vi "SEVEN SEGMENT DISPLAY FROM 0-25.vi"() -> ()   [LabVIEW 2019]
panel:
  in  "STOP":bool
  in  "NUMBER":u8
  out "E 2":bool
  out "D 2":bool
  out "C 2":bool
  out "F 2":bool
  out "G 2":bool
  out "B 2":bool
  out "A 2":bool
  out "E":bool
  out "D":bool
  out "C":bool
  out "F":bool
  out "G":bool
  out "B":bool
  out "A":bool
  # "SEVEN SEGMENT DISPLAY FROM 0-25"
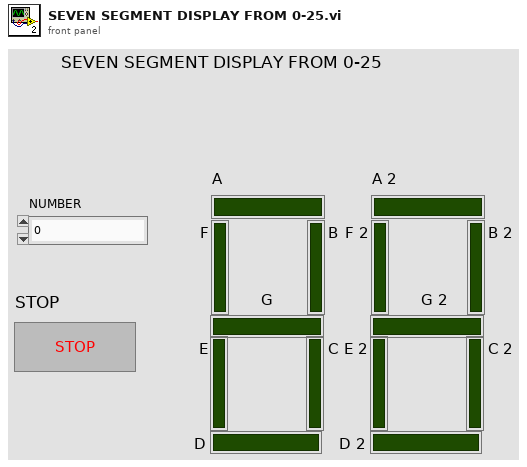
[diagram p1: front panel]
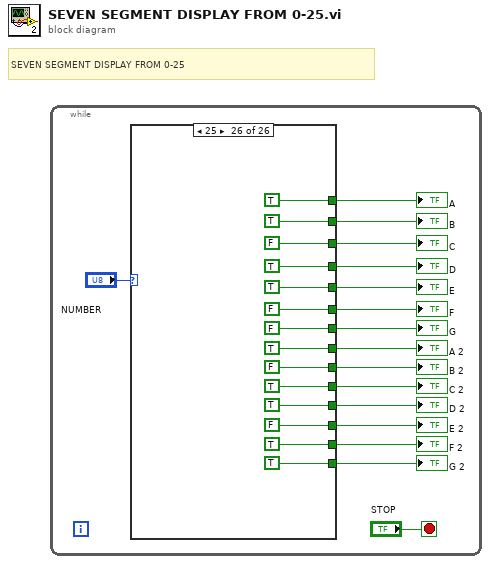
[diagram p0: block diagram]
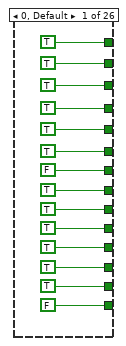
[diagram p2: hidden frame]
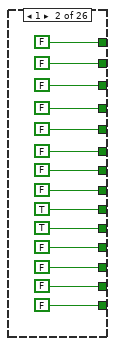
[diagram p3: hidden frame]
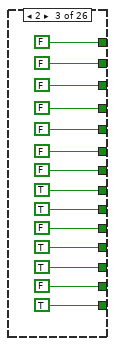
[diagram p4: hidden frame]
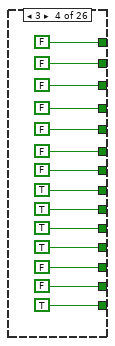
[diagram p5: hidden frame]
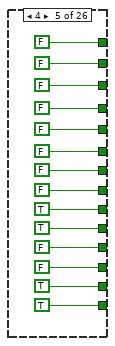
[diagram p6: hidden frame]
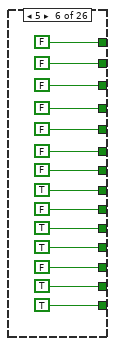
[diagram p7: hidden frame]
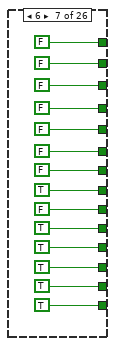
[diagram p8: hidden frame]
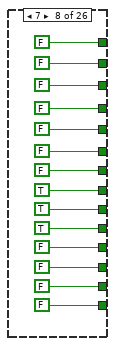
[diagram p9: hidden frame]
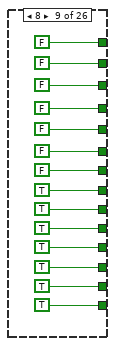
[diagram p10: hidden frame]
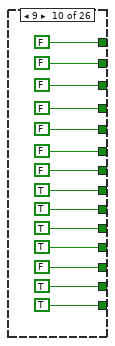
[diagram p11: hidden frame]
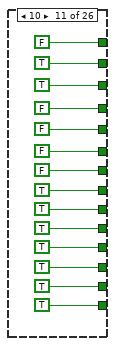
[diagram p12: hidden frame]
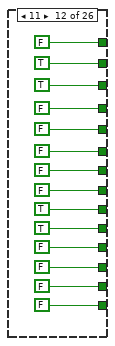
[diagram p13: hidden frame]
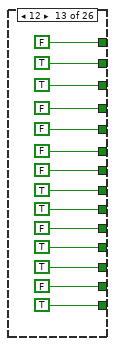
[diagram p14: hidden frame]
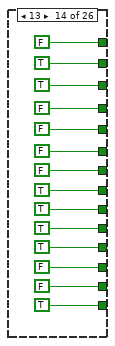
[diagram p15: hidden frame]
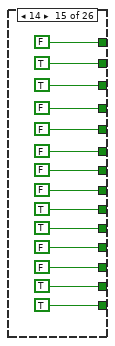
[diagram p16: hidden frame]
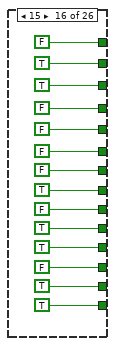
[diagram p17: hidden frame]
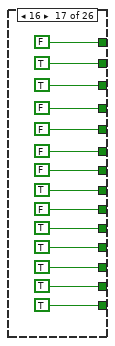
[diagram p18: hidden frame]
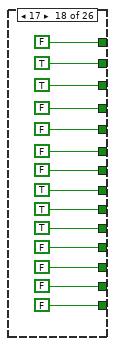
[diagram p19: hidden frame]
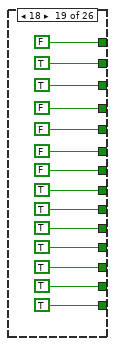
[diagram p20: hidden frame]
diagram:
  # "SEVEN SEGMENT DISPLAY FROM 0-25"
  n1 = while {
    stop <- "STOP" stop-if-true
    n2 = case shown="25" "NUMBER" {
      tunnel: [TRUE ("A") FALSE ("A") FALSE ("A") FALSE ("A") FALSE ("A") FALSE ("A") FALSE ("A") FALSE ("A") FALSE ("A") FALSE ("A") FALSE ("A") FALSE ("A") FALSE ("A") FALSE ("A") FALSE ("A") FALSE ("A") FALSE ("A") FALSE ("A") FALSE ("A") FALSE ("A") TRUE ("A") TRUE ("A") TRUE ("A") TRUE ("A") TRUE ("A") TRUE ("A")] -> w16
      tunnel: [FALSE ("G") FALSE ("G") FALSE ("G") FALSE ("G") FALSE ("G") FALSE ("G") FALSE ("G") FALSE ("G") FALSE ("G") FALSE ("G") FALSE ("G") FALSE ("G") FALSE ("G") FALSE ("G") FALSE ("G") FALSE ("G") FALSE ("G") FALSE ("G") FALSE ("G") FALSE ("G") TRUE ("G") FALSE ("G") FALSE ("G") FALSE ("G") FALSE ("G") FALSE ("G")] -> w15
      tunnel: [TRUE ("F") FALSE ("F") FALSE ("F") FALSE ("F") FALSE ("F") FALSE ("F") FALSE ("F") FALSE ("F") FALSE ("F") FALSE ("F") FALSE ("F") FALSE ("F") FALSE ("F") FALSE ("F") FALSE ("F") FALSE ("F") FALSE ("F") FALSE ("F") FALSE ("F") FALSE ("F") FALSE ("F") FALSE ("F") FALSE ("F") FALSE ("F") FALSE ("F") FALSE ("F")] -> w14
      tunnel: [TRUE ("C") FALSE ("C") FALSE ("C") FALSE ("C") FALSE ("C") FALSE ("C") FALSE ("C") FALSE ("C") FALSE ("C") FALSE ("C") TRUE ("C") TRUE ("C") TRUE ("C") TRUE ("C") TRUE ("C") TRUE ("C") TRUE ("C") TRUE ("C") TRUE ("C") TRUE ("C") FALSE ("C") FALSE ("C") FALSE ("C") FALSE ("C") FALSE ("C") FALSE ("C")] -> w13
      tunnel: [TRUE ("D") FALSE ("D") FALSE ("D") FALSE ("D") FALSE ("D") FALSE ("D") FALSE ("D") FALSE ("D") FALSE ("D") FALSE ("D") FALSE ("D") FALSE ("D") FALSE ("D") FALSE ("D") FALSE ("D") FALSE ("D") FALSE ("D") FALSE ("D") FALSE ("D") FALSE ("D") TRUE ("D") TRUE ("D") TRUE ("D") TRUE ("D") TRUE ("D") TRUE ("D")] -> w12
      tunnel: [TRUE ("E") FALSE ("E") FALSE ("E") FALSE ("E") FALSE ("E") FALSE ("E") FALSE ("E") FALSE ("E") FALSE ("E") FALSE ("E") FALSE ("E") FALSE ("E") FALSE ("E") FALSE ("E") FALSE ("E") FALSE ("E") FALSE ("E") FALSE ("E") FALSE ("E") FALSE ("E") TRUE ("E") TRUE ("E") TRUE ("E") TRUE ("E") TRUE ("E") TRUE ("E")] -> w11
      tunnel: [TRUE ("A 2") FALSE ("A 2") TRUE ("A 2") TRUE ("A 2") FALSE ("A 2") TRUE ("A 2") TRUE ("A 2") TRUE ("A 2") TRUE ("A 2") TRUE ("A 2") TRUE ("A 2") FALSE ("A 2") TRUE ("A 2") TRUE ("A 2") FALSE ("A 2") TRUE ("A 2") TRUE ("A 2") TRUE ("A 2") TRUE ("A 2") TRUE ("A 2") TRUE ("A 2") FALSE ("A 2") TRUE ("A 2") TRUE ("A 2") FALSE ("A 2") TRUE ("A 2")] -> w10
      tunnel: [TRUE ("B 2") TRUE ("B 2") TRUE ("B 2") TRUE ("B 2") TRUE ("B 2") FALSE ("B 2") FALSE ("B 2") TRUE ("B 2") TRUE ("B 2") TRUE ("B 2") TRUE ("B 2") TRUE ("B 2") TRUE ("B 2") TRUE ("B 2") TRUE ("B 2") FALSE ("B 2") FALSE ("B 2") TRUE ("B 2") TRUE ("B 2") TRUE ("B 2") TRUE ("B 2") TRUE ("B 2") TRUE ("B 2") TRUE ("B 2") TRUE ("B 2") FALSE ("B 2")] -> w9
      tunnel: [FALSE ("G 2") FALSE ("G 2") TRUE ("G 2") TRUE ("G 2") TRUE ("G 2") TRUE ("G 2") TRUE ("G 2") FALSE ("G 2") TRUE ("G 2") TRUE ("G 2") TRUE ("G 2") FALSE ("G 2") TRUE ("G 2") TRUE ("G 2") TRUE ("G 2") TRUE ("G 2") TRUE ("G 2") FALSE ("G 2") TRUE ("G 2") TRUE ("G 2") FALSE ("G 2") FALSE ("G 2") FALSE ("G 2") TRUE ("G 2") TRUE ("G 2") TRUE ("G 2")] -> w8
      tunnel: [TRUE ("F 2") FALSE ("F 2") FALSE ("F 2") FALSE ("F 2") TRUE ("F 2") TRUE ("F 2") TRUE ("F 2") FALSE ("F 2") TRUE ("F 2") TRUE ("F 2") TRUE ("F 2") FALSE ("F 2") FALSE ("F 2") FALSE ("F 2") TRUE ("F 2") TRUE ("F 2") TRUE ("F 2") FALSE ("F 2") TRUE ("F 2") TRUE ("F 2") TRUE ("F 2") FALSE ("F 2") FALSE ("F 2") FALSE ("F 2") TRUE ("F 2") TRUE ("F 2")] -> w7
      tunnel: [TRUE ("C 2") TRUE ("C 2") FALSE ("C 2") TRUE ("C 2") TRUE ("C 2") TRUE ("C 2") TRUE ("C 2") TRUE ("C 2") TRUE ("C 2") TRUE ("C 2") TRUE ("C 2") TRUE ("C 2") FALSE ("C 2") TRUE ("C 2") TRUE ("C 2") TRUE ("C 2") TRUE ("C 2") TRUE ("C 2") TRUE ("C 2") TRUE ("C 2") TRUE ("C 2") TRUE ("C 2") FALSE ("C 2") TRUE ("C 2") TRUE ("C 2") TRUE ("C 2")] -> w6
      tunnel: [TRUE ("D 2") FALSE ("D 2") TRUE ("D 2") TRUE ("D 2") FALSE ("D 2") TRUE ("D 2") TRUE ("D 2") FALSE ("D 2") TRUE ("D 2") TRUE ("D 2") TRUE ("D 2") FALSE ("D 2") TRUE ("D 2") TRUE ("D 2") FALSE ("D 2") TRUE ("D 2") TRUE ("D 2") FALSE ("D 2") TRUE ("D 2") TRUE ("D 2") TRUE ("D 2") FALSE ("D 2") TRUE ("D 2") TRUE ("D 2") FALSE ("D 2") TRUE ("D 2")] -> w5
      tunnel: [TRUE ("E 2") FALSE ("E 2") TRUE ("E 2") FALSE ("E 2") FALSE ("E 2") FALSE ("E 2") TRUE ("E 2") FALSE ("E 2") TRUE ("E 2") FALSE ("E 2") TRUE ("E 2") FALSE ("E 2") TRUE ("E 2") FALSE ("E 2") FALSE ("E 2") FALSE ("E 2") TRUE ("E 2") FALSE ("E 2") TRUE ("E 2") FALSE ("E 2") TRUE ("E 2") FALSE ("E 2") TRUE ("E 2") FALSE ("E 2") FALSE ("E 2") FALSE ("E 2")] -> w4
      tunnel: [TRUE ("B") FALSE ("B") FALSE ("B") FALSE ("B") FALSE ("B") FALSE ("B") FALSE ("B") FALSE ("B") FALSE ("B") FALSE ("B") TRUE ("B") TRUE ("B") TRUE ("B") TRUE ("B") TRUE ("B") TRUE ("B") TRUE ("B") TRUE ("B") TRUE ("B") TRUE ("B") TRUE ("B") TRUE ("B") TRUE ("B") TRUE ("B") TRUE ("B") TRUE ("B")] -> w3
      frame 0, Default {
      }
      frame 1 {
      }
      frame 2 {
      }
      frame 3 {
      }
      frame 4 {
      }
      frame 5 {
      }
      frame 6 {
      }
      frame 7 {
      }
      frame 8 {
      }
      frame 9 {
      }
      frame 10 {
      }
      frame 11 {
      }
      frame 12 {
      }
      frame 13 {
      }
      frame 14 {
      }
      frame 15 {
      }
      frame 16 {
      }
      frame 17 {
      }
      frame 18 {
      }
      frame 19 {
      }
      frame 20 {
      }
      frame 21 {
      }
      frame 22 {
      }
      frame 23 {
      }
      frame 24 {
      }
      frame 25 {
      }
    }
    "A 2" <- w10
    "B 2" <- w9
    "G 2" <- w8
    "F 2" <- w7
    "C 2" <- w6
    "D 2" <- w5
    "E 2" <- w4
    "A" <- w16
    "B" <- w3
    "G" <- w15
    "F" <- w14
    "C" <- w13
    "D" <- w12
    "E" <- w11
  }
